vi "Handle.vi"(8 "error in (no error)":errorcluster, 11 "WeatherStation in":refnum<class "WeatherStation.lvclass">) -> (0 "error out":errorcluster, 3 "WeatherStation out":refnum<class "WeatherStation.lvclass">)   [LabVIEW 2018, in "WeatherStation.lvclass"]
uses:
  WeatherStation.lvclass
  WeatherStation.lvclass/WeatherStation.ctl
  Device/Device.lvclass/Device.ctl
  WeatherSensor/WeatherSensor.lvclass
  C:/Users/observer/Desktop/Sparc4GUI/Versao ZeroMQ/SPARC4_GUI -20240711_20240708/Device/Device.lvclass
  Server/Server.lvclass
  Comm/Stream/Stream.lvclass
  Device/Device.lvclass
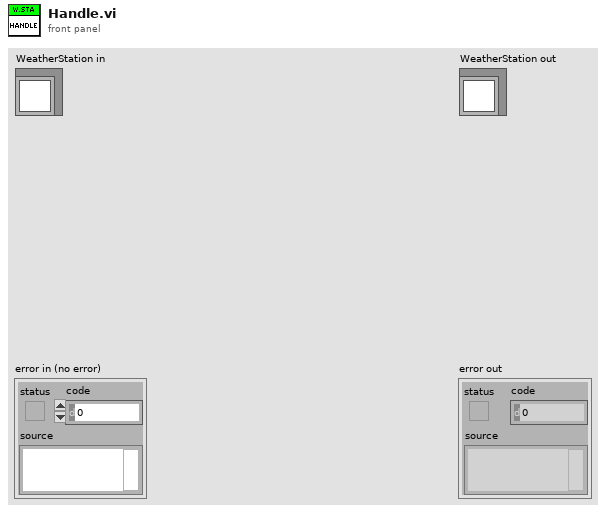
[diagram p1: front panel]
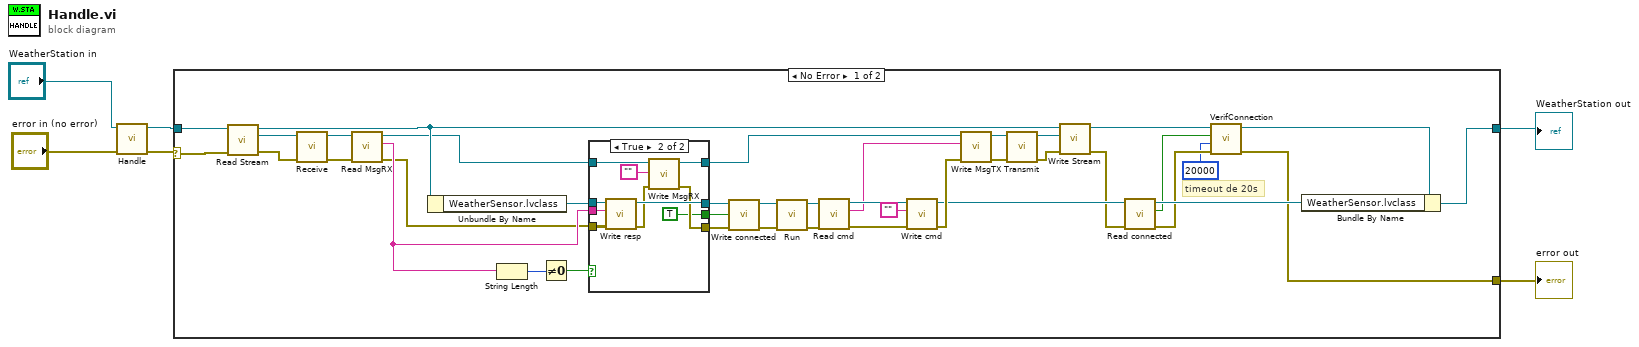
[diagram p0: block diagram]
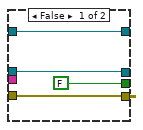
[diagram p2: hidden frame]
diagram:
  n1 = call-parent "Handle.vi"("error in (no error)"="error in (no error)", "Server in"="WeatherStation in") -> ("error out"=w3:errorcluster, "Server out"=w4:refnum<class "WeatherStation.lvclass">)  [unwired: 8 in]
  n2 = case shown="No Error" w3 {
    selector: w3 -> [w44 w62]
    tunnel: [w19 w62] -> w2
    tunnel: [w43 w61] -> w1
    tunnel: w4 -> [w36 w61]
    frame No Error {
      # "timeout de 20s"
      n3 = call-dynamic "Read Stream.vi"("error in (no error)"=w44, "Server in"=w36) -> ("error out"=w45:errorcluster, "Stream.lvclass"=w46:refnum<class "Stream.lvclass">, "Server out"=w17:refnum<class "WeatherStation.lvclass">)  [unwired: 7 in]
      n4 = call-dynamic "Receive.vi"("error in (no error)"=w45, "Stream in"=w46) -> ("error out"=w42:errorcluster, "Stream out"=w41:refnum<class "Stream.lvclass">)  [unwired: 8 in]
      n5 = call-dynamic "Read MsgRX.vi"("error in (no error)"=w42, "Comm in"=w41) -> ("error out"=w14:errorcluster, "MsgRX"=w15:string, "Comm out"=w9:refnum<class "Stream.lvclass">)  [unwired: 7 in]
      n6 = Unbundle By Name(w17) -> ("WeatherSensor.lvclass"=w16:refnum<class "WeatherSensor.lvclass">)
      n7 = String Length(string=w15) -> (length=w30:i32)
      n8 = Not Equal To 0?(x=w30) -> (x != 0?=w29:bool)
      n9 = case shown="True" w29 {
        tunnel: [w49 w53] -> w11
        tunnel: [w50 w59] -> w13
        tunnel: w14 -> [w49 w57]
        tunnel: w16 -> [w50 w60]
        tunnel: w15 -> [_ w58]
        tunnel: w9 -> [w47 w56]
        tunnel: [w47 w55] -> w8
        tunnel: [FALSE TRUE] -> w7
        frame False {
        }
        frame True {
          n10 = call-dynamic "Write resp.vi"("error in (no error)"=w57, "resp"=w58, "Device in"=w60) -> ("error out"=w54:errorcluster, "Device out"=w59:refnum<class "WeatherSensor.lvclass">)  [unwired: 7 in]
          n11 = call-dynamic "Write MsgRX.vi"("error in (no error)"=w54, "MsgRX"="", "Comm in"=w56) -> ("error out"=w53:errorcluster, "Comm out"=w55:refnum<class "Stream.lvclass">)  [unwired: 7 in]
        }
      }
      n12 = call "Write connected.vi"("error in (no error)"=w11, "connected"=w7, "Device in"=w13) -> ("error out"=w10:errorcluster, "Device out"=w12:refnum<class "WeatherSensor.lvclass">)  [unwired: 7 in]
      n13 = call-dynamic "Run.vi"("error in (no error)"=w10, "WeatherSensor in"=w12) -> ("error out"=w27:errorcluster, "WeatherSensor out"=w28:refnum<class "WeatherSensor.lvclass">)  [unwired: 8 in]
      n14 = call-dynamic "Read cmd.vi"("error in (no error)"=w27, "Device in"=w28) -> ("error out"=w34:errorcluster, "cmd"=w32:string, "Device out"=w35:refnum<class "WeatherSensor.lvclass">)  [unwired: 7 in]
      n15 = call-dynamic "Write cmd.vi"("error in (no error)"=w34, "cmd"="", "Device in"=w35) -> ("error out"=w40:errorcluster, "Device out"=w26:refnum<class "WeatherSensor.lvclass">)  [unwired: 7 in]
      n16 = call-dynamic "Write MsgTX.vi"("error in (no error)"=w40, "MsgTX"=w32, "Comm in"=w8) -> ("error out"=w38:errorcluster, "Comm out"=w39:refnum<class "Stream.lvclass">)  [unwired: 7 in]
      n17 = call-dynamic "Transmit.vi"("error in (no error)"=w38, "Stream in"=w39) -> ("error out"=w37:errorcluster, "Stream out"=w31:refnum<class "Stream.lvclass">)  [unwired: 8 in]
      n18 = call-dynamic "Write Stream.vi"("error in (no error)"=w37, "Stream.lvclass"=w31, "Server in"=w17) -> ("error out"=w25:errorcluster, "Server out"=w24:refnum<class "WeatherStation.lvclass">)  [unwired: 7 in]
      n19 = call "Read connected.vi"("error in (no error)"=w25, "Device in"=w26) -> ("error out"=w20:errorcluster, "connected"=w22:bool, "Device out"=w23:refnum<class "WeatherSensor.lvclass">)  [unwired: 7 in]
      n20 = call-dynamic "VerifConnection.vi"("error in (no error)"=w20, "timeout in ms (1000)"=u32 20000 ("period (ms)"), "device connected in"=w22, "Server in"=w24) -> ("error out"=w19:errorcluster, "Server out"=w21:refnum<class "WeatherStation.lvclass">)  [unwired: 6 in]
      n21 = Bundle By Name(cluster=w21, "WeatherSensor.lvclass"=w23) -> (w43:refnum<class "WeatherStation.lvclass">)
    }
    frame Error {
    }
  }
  "error out" <- w2
  "WeatherStation out" <- w1
